vi "Read FPGA Ref.vi"(8 "error in (no error)":errorcluster, 11 "FPGA Session in":refnum<class "FPGA Session.lvclass">) -> (0 "error out":errorcluster, 2 "FPGA Ref":T1, 3 "FPGA Session out":refnum<class "FPGA Session.lvclass">)   [LabVIEW 2017, in "FPGA Session.lvclass"]
uses:
  FPGA Session.lvclass
  FPGA Ref.ctl
  FPGA Session.lvclass/FPGA Session.ctl
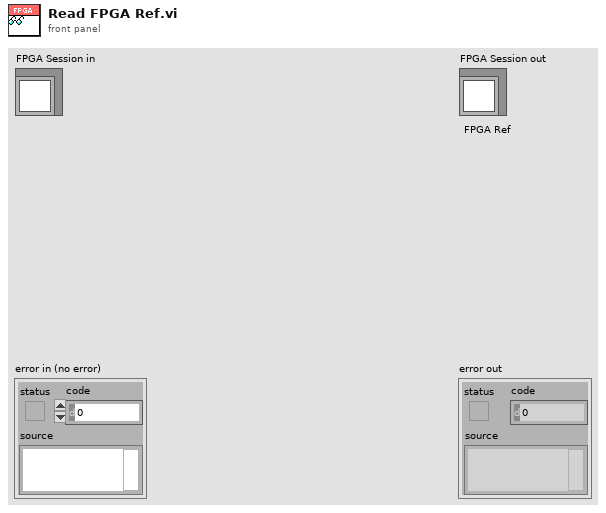
[diagram p1: front panel]
types:
  T1 = typedef "FPGA Ref.ctl" = refnum<k20>
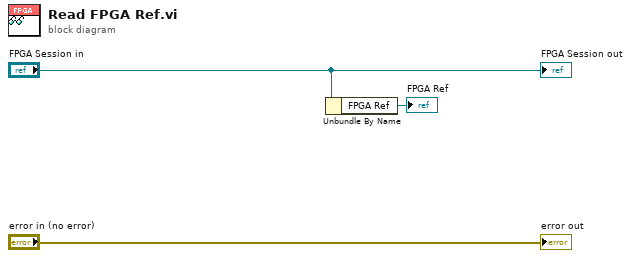
[diagram p0: block diagram]
diagram:
  n1 = Unbundle By Name("FPGA Session in") -> ("FPGA Ref"=→"FPGA Ref":T1)
  "error out" <- "error in (no error)"
  "FPGA Session out" <- "FPGA Session in"
